vi "SCC Compare Files.vi"(4 "version":string, 6 "compare options":T1, 7 "advanced options":variant, 8 "error in (no error)":errorcluster, 9 "compare method":T2 items=["source control provider default", "contents (silent)", "checksum (silent)", "time (silent)"], 10 "file path":path, 11 "source control reference in":T3) -> (0 "error out":errorcluster, 2 "status message":string, 3 "source control reference out":T3, 5 "file differs?":bool)   [LabVIEW 2017, in "NI_SCC.lvlib"]
doc: "Returns the difference between the specified file and, by default, the latest version of the file in source control."
uses:
  <vilib>/SourceControl/sccapi/NI_SCC.lvlib
  <vilib>/SourceControl/sccapi/SCCAPI Refnum.ctl
  <vilib>/SourceControl/sccapi/SCCAPI Compare Method.ctl
  <vilib>/SourceControl/sccapi/SCCAPI Compare Options.ctl
  <vilib>/SourceControl/sccapi/SCCAPI SCC Operations.ctl
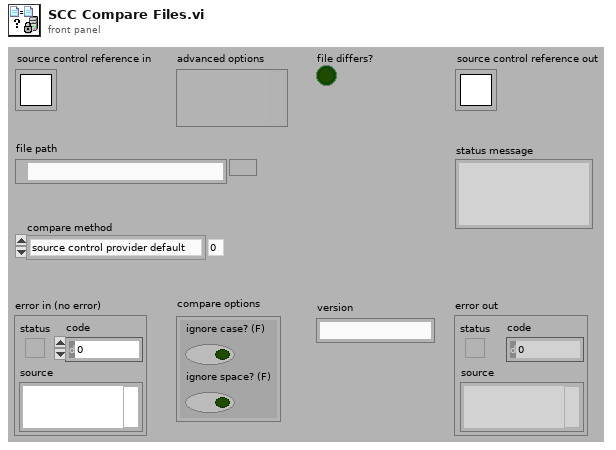
[diagram p1: front panel]
types:
  T1 = typedef "NI_SCC.lvlib/SCCAPI Compare Options.ctl" = cluster{"ignore case? (F)":bool, "ignore space? (F)":bool}
  T2 = typedef "NI_SCC.lvlib/SCCAPI Compare Method.ctl" = u16
  T3 = typedef "NI_SCC.lvlib/SCCAPI Refnum.ctl" = refnum<k1>
  T4 = typedef "NI_SCC.lvlib/SCCAPI SCC Operations.ctl" = enum16{"Add", "Check In", "Check Out", "Close Project", "Compare Files", "Compare VIs", "Configure Project", "File History", "File Properties", "File Status", "Find All Providers", "Get Advanced Command Options", "Get File Copy", "Get Latest Version", "Get Project Name", "Get StaticVI Path", "Initialize", "Not A Source Control Reference", "Open Project", "Provider Supports Functionality", "Remove", "Run Provider", "Undo Check Out", "Uninitialize", "Is File In Local Path"}
  T5 = typedef "SCCAPI Refnum.ctl" = refnum<k1>
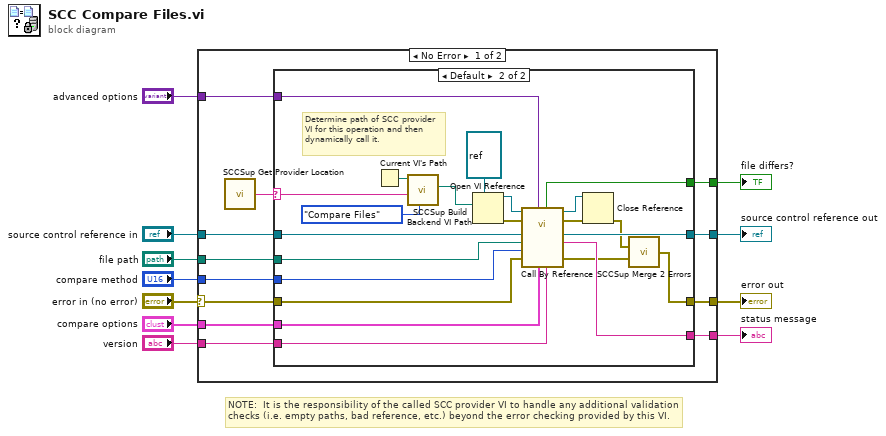
[diagram p0: block diagram]
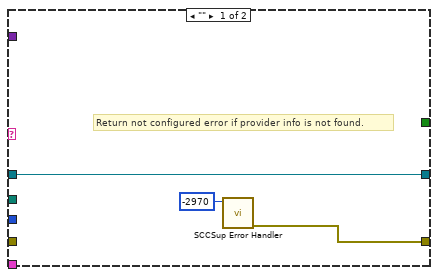
[diagram p2: hidden frame]
diagram:
  # "NOTE:  It is the responsibility of the called SCC provider VI to handle any additional validation checks (i.e. empty paths, bad reference, etc.) beyond the error checking provided by this VI."
  n1 = case shown="No Error" "error in (no error)" {
    selector: "error in (no error)" -> [w15 w50]
    tunnel: [w23 w50] -> w10
    tunnel: "source control reference in" -> [w22 w49]
    tunnel: [w21 _] -> w8
    tunnel: [w20 w49] -> w7
    tunnel: "file path" -> [w19 _]
    tunnel: "compare method" -> [w18 _]
    tunnel: [w17 _] -> w4
    tunnel: "advanced options" -> [w14 _]
    tunnel: "compare options" -> [w13 _]
    tunnel: "version" -> [w12 _]
    frame No Error {
      n2 = call <vilib>:"SCCSup Get Provider Location.vi"() -> ("provider location"=w16:string)  [unwired: 6 in]
      n3 = case shown="Default" w16 {
        selector: w16 -> [_ w31]
        tunnel: [w24 w48] -> w23
        tunnel: w22 -> [w26 w40]
        tunnel: [_ w47] -> w21
        tunnel: [w26 w41] -> w20
        tunnel: w19 -> [_ w39]
        tunnel: w18 -> [_ w38]
        tunnel: [_ w37] -> w17
        tunnel: w15 -> [_ w30]
        tunnel: w14 -> [_ w29]
        tunnel: w13 -> [_ w28]
        tunnel: w12 -> [_ w27]
        frame "" {
          # "Return not configured error if provider info is not found."
          n4 = call <vilib>:"SCCSup Error Handler.vi"("scc error code"=-2970 ("code")) -> ("error out"=w24:errorcluster)  [unwired: 10 in]
        }
        frame Default {
          # "Determine path of SCC provider VI for this operation and then dynamically call it."
          n5 = Current VI's Path() -> (path=w34:path)
          n6 = call <vilib>:"SCCSup Build Backend VI Path.vi"("scc operation"=SCCAPI_SCC_Operations."Compare Files", "provider location"=w31, "caller path"=w34) -> ("scc backend VI path"=w33:path)  [unwired: 8 in]
          n7 = Open VI Reference(type specifier VI Refnum (for type only)=refnum<vi> refnum, vi path=w33) -> (vi reference=w45:refnum<vi>, error out=w44:errorcluster)  [unwired: 4 in]
          n8 = call-by-ref "?"(reference=w45, error in=w44, "version"=w27, "compare options"=w28, "advanced options"=w29, "error in (no error)"=w30, "compare method"=w38, "filename"=w39, "source control reference in"=w40) -> (reference out=w43:refnum<vi>, error out=w42:errorcluster, 0:"error out"=w35:errorcluster, "status message"=w47:string, "source control reference out"=w41:T5, "file differs?"=w37:bool)  [unwired: 1 in]
          n9 = Close Reference(reference=w43, error in (no error)=w42) -> (error out=w36:errorcluster)
          n10 = call <vilib>:"SCCSup Merge 2 Errors.vi"("Error IO 1"=w36, "Error IO 2"=w35) -> ("Error IO out"=w48:errorcluster)  [unwired: 13 in]
        }
      }
    }
    frame Error {
    }
  }
  "error out" <- w10
  "status message" <- w8
  "source control reference out" <- w7
  "file differs?" <- w4
